vi "Array_Min_Batch(CuLab).vi"(6 "operation":enum16{"avg", "min", "max", "maxmin"}(ring)=enum."min", 8 "error in":errorcluster, 11 "T2D_SGL out":refnum<class "T2D_SGL.lvclass">) -> (0 "error out":errorcluster, 3 "T1D_SGL out":refnum<class "T1D_SGL.lvclass">)   [LabVIEW 2020, in "PatchCore_AddOn.lvlib"]
uses:
  PatchCore_AddOn.lvlib
  <vilib>/Ngene/CuLab - GPU Accelerated Toolkit/Toolkit/Low_Level/Tensor_Classes/T_Children/T2D/T2D_Children/T2D_SGL/T2D_SGL.lvclass
  C:/Program Files/National Instruments/LabVIEW 2020/vi.lib/Ngene/CuLab - GPU Accelerated Toolkit/Toolkit/Low_Level/Tensor_Classes/T_Children/T2D/T2D.lvclass
  <vilib>/Ngene/CuLab - GPU Accelerated Toolkit/Toolkit/Low_Level/Tensor_Classes/T_Children/T1D/T1D_Children/T1D_SGL/T1D_SGL.lvclass
  C:/Program Files/National Instruments/LabVIEW 2020/vi.lib/Ngene/CuLab - GPU Accelerated Toolkit/Toolkit/Low_Level/Tensor_Classes/T_Children/T1D/T1D.lvclass
  <vilib>/Ngene/CuLab - GPU Accelerated Toolkit/Toolkit/Low_Level/Tensor_Classes/T_Children/T1D/Controls/T1D_Dims.ctl
  <vilib>/Ngene/CuLab - GPU Accelerated Toolkit/Toolkit/Low_Level/Tensor_Classes/T_Children/T2D/Controls/T2D_Dims.ctl
  <vilib>/Ngene/CuLab - GPU Accelerated Toolkit/Toolkit/Low_Level/Tensor_Classes/T_Children/T2D/Controls/T2D_Indices.ctl
  <vilib>/Ngene/CuLab - GPU Accelerated Toolkit/Toolkit/API/Array/Array Size/CU_Array_Size_T2D.vi
  <vilib>/Ngene/CuLab - GPU Accelerated Toolkit/Toolkit/API/Array/Replace Array Subset (API)/CU_Replace_Array_Subset_1D_1D/CU_Replace_Array_Subset_1D_1D_SGL.vi
  <vilib>/Ngene/CuLab - GPU Accelerated Toolkit/Toolkit/API/Array/Array Subset/T2D/CU_Array_Subset_T2D_SGL.vi
  <vilib>/Ngene/CuLab - GPU Accelerated Toolkit/Toolkit/API/Signal Processing/Signal Operation/Decimate (single shot) adaptive/CU_Decimate_Single_Shot_Adaptive_T1D_SGL.vi
  <vilib>/Ngene/CuLab - GPU Accelerated Toolkit/Toolkit/API/Array/Reshape Array  (API)/CU_Reshape_to_T1D/T2D/CU_Reshape_to_T1D_(T2D_SGL).vi
  <vilib>/Ngene/CuLab - GPU Accelerated Toolkit/Toolkit/CuLab.lvlib
  C:/Program Files/National Instruments/LabVIEW 2020/vi.lib/Ngene/CuLab - GPU Accelerated Toolkit/Toolkit/Low_Level/Tensor_Classes/Tensor.lvclass
  C:/Program Files/National Instruments/LabVIEW 2020/vi.lib/Ngene/CuLab - GPU Accelerated Toolkit/Toolkit/Low_Level/Tensor_Classes/T_Children/T2D/T2D_Children/T2D_SGL/T2D_SGL.lvclass
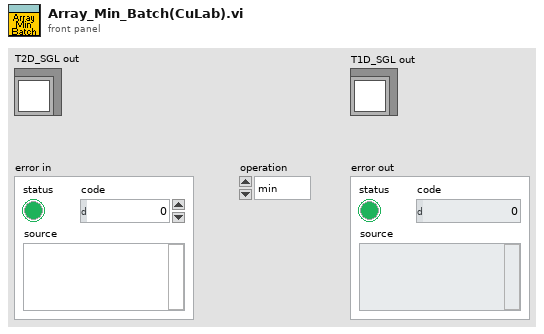
[diagram p1: front panel]
types:
  T1 = typedef "CuLab.lvlib/T1D_Dims.ctl" = cluster{"W":i32}
  T2 = typedef "CuLab.lvlib/T2D_Dims.ctl" = cluster{"H":i32, "W":i32}
  T3 = typedef "CuLab.lvlib/T2D_Indices.ctl" = cluster{"i":i32, "j":i32}
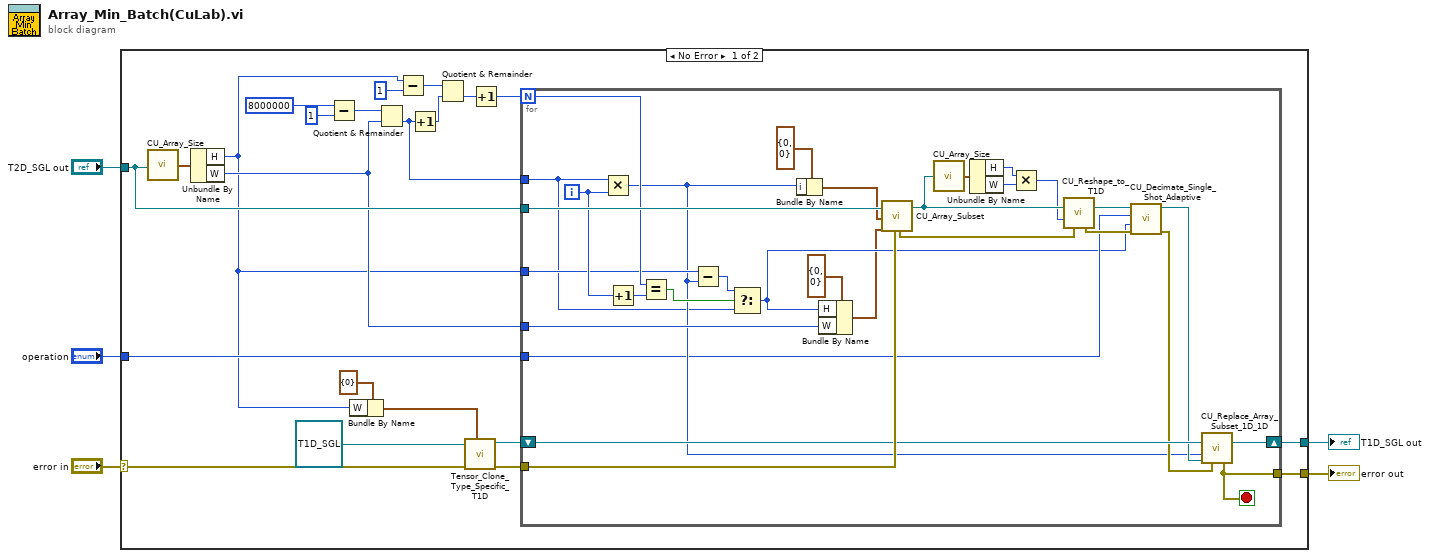
[diagram p0: block diagram]
diagram:
  n1 = case shown="No Error" "error in" {
    selector: "error in" -> [w25 w58]
    tunnel: "T2D_SGL out" -> [w24 _]
    tunnel: "operation" -> [w27 _]
    tunnel: [w26 w58] -> w2
    tunnel: [w23 _] -> w1
    frame No Error {
      n2 = call-poly <vilib>:"CU_Array_Size.vi"("Tensor"=w24) -> ("T2D_Dims"=w22:T2)  [unwired: 14 in]
      n3 = Unbundle By Name(w22) -> ("H"=w8:i32, "W"=w10:i32)
      n4 = Subtract(x=8000000 ("y"), y=1) -> (x-y=w15:i32)
      n5 = Bundle By Name(cluster=T1 {"W"=0} ("Dest_Tensor_Dims"), "W"=w8) -> (w19:T1)
      n6 = Quotient & Remainder(x=w15, y=w10) -> (floor(x/y)=w6:i32)  [unwired: 1 out]
      n7 = Subtract(x=w8, y=1) -> (x-y=w12:i32)
      n8 = Increment(x=w6) -> (x+1=w7:i32)
      n9 = Quotient & Remainder(x=w12, y=w7) -> (floor(x/y)=w13:i32)  [unwired: 1 out]
      n10 = call <vilib>:"Tensor_Clone_Type_Specific_T1D.vi"("Dest_Tensor_Dims"=w19, "error in (no error)"=w25, "Dest_Tensor"=refnum<class "T1D_SGL.lvclass"> refnum ("pred score")) -> ("error out"=w17:errorcluster, "Dest_Tensor out"=w18:refnum<class "T1D_SGL.lvclass">)  [unwired: 7 in]
      n11 = Increment(x=w13) -> (x+1=w9:i32)
      n12 = for {
        N: w9 -> [w40]
        tunnel: w24 -> [w57]
        tunnel: w27 -> [w31]
        tunnel: w8 -> [w38]
        shift-right: [w37] -> w23
        shift-left: w18 -> [w45]
        tunnel: w17 -> [w56]
        tunnel: [w35] -> w26
        tunnel: w10 -> [w39]
        tunnel: w6 -> [w28]
        i -> [w44]
        stop <- w35 stop-if-true
        n13 = Multiply(x=w28, y=w44) -> (x*y=w33:i32)
        n14 = Increment(x=w44) -> (x+1=w43:i32)
        n15 = Equal?(x=w40, y=w43) -> (x = y?=w42:bool)
        n16 = Subtract(x=w38, y=w33) -> (x-y=w41:i32)
        n17 = Select(t=w41, s=w42, f=w28) -> (s? t:f=w30:i32)
        n18 = Bundle By Name(cluster=T3 {"i"=0, "j"=0} ("Indices"), "i"=w33) -> (w32:T3)
        n19 = Bundle By Name(cluster=T2 {"H"=0, "W"=0} ("Lengths"), "H"=w30, "W"=w39) -> (w29:T2)
        n20 = call-poly <vilib>:"CU_Array_Subset.vi"("Tensor in"=w57, "Indices"=w32, "Lengths"=w29, "error in (no error)"=w56) -> ("error out"=w47:errorcluster, "Dest out"=w53:refnum<class "T2D_SGL.lvclass">)  [unwired: 14 in]
        n21 = call-poly <vilib>:"CU_Array_Size.vi"("Tensor"=w53) -> ("T2D_Dims"=w52:T2)  [unwired: 14 in]
        n22 = Unbundle By Name(w52) -> ("H"=w51:i32, "W"=w50:i32)
        n23 = Multiply(x=w51, y=w50) -> (x*y=w49:i32)
        n24 = call-poly <vilib>:"CU_Reshape_to_T1D.vi"("Tensor in"=w53, "Dest Dim"=w49, "error in (no error)"=w47) -> ("Dest out"=w48:refnum<class "T1D_SGL.lvclass">, "error out"=w46:errorcluster)  [unwired: 11 in]
        n25 = call-poly <vilib>:"CU_Decimate_Single_Shot_Adaptive.vi"("error in (no error)"=w46, "output size"=w30, "operation"=w31, "X"=w48) -> ("error out"=w36:errorcluster, "Y"=w34:refnum<class "T1D_SGL.lvclass">)  [unwired: 6 in]
        n26 = call-poly <vilib>:"CU_Replace_Array_Subset_1D_1D.vi"("Tensor in"=w45, "index"=w33, "Sub Tensor"=w34, "error in (no error)"=w36) -> ("Tensor Out"=w37:refnum<class "T1D_SGL.lvclass">, "error out"=w35:errorcluster)  [unwired: 10 in]
      }
    }
    frame Error {
    }
  }
  "error out" <- w2
  "T1D_SGL out" <- w1
